vi "Input_Sync_1.vi"(0 "Delay":dbl, 5 "SampClk.Timebase.Rate in":dbl) -> (2 "SampClk.Timebase.Rate 3":dbl, 3 "task out":refnum<k21>, 4 "Refnum out":refnum<k21>, 6 "SampClk.Rate 2":dbl, 8 "error out 2":errorcluster, 10 "FirstSampClkWhen":timestamp, 13 "SampClk.Timebase.Rate out":dbl, 14 "SampClk.Rate":dbl, 15 "error out":errorcluster)   [LabVIEW 2020]
uses:
  <vilib>/DAQmx/create/channels.llb/DAQmx Create Channel (AI-Voltage-Basic).vi
  <vilib>/DAQmx/create/channels.llb/DAQmx Create Channel (TEDS-AI-Voltage-Basic).vi
  <vilib>/DAQmx/configure/timing.llb/DAQmx Timing (Sample Clock).vi
  <vilib>/DAQmx/create/channels.llb/DAQmx Create Channel (AI-Temperature-Thermocouple).vi
  <resource>/objmgr/daqmx.rc
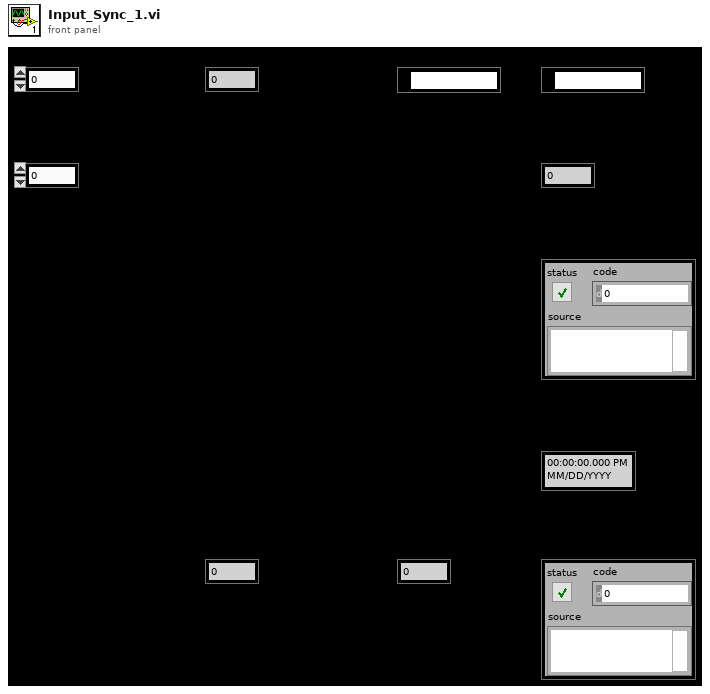
[diagram p1: front panel]
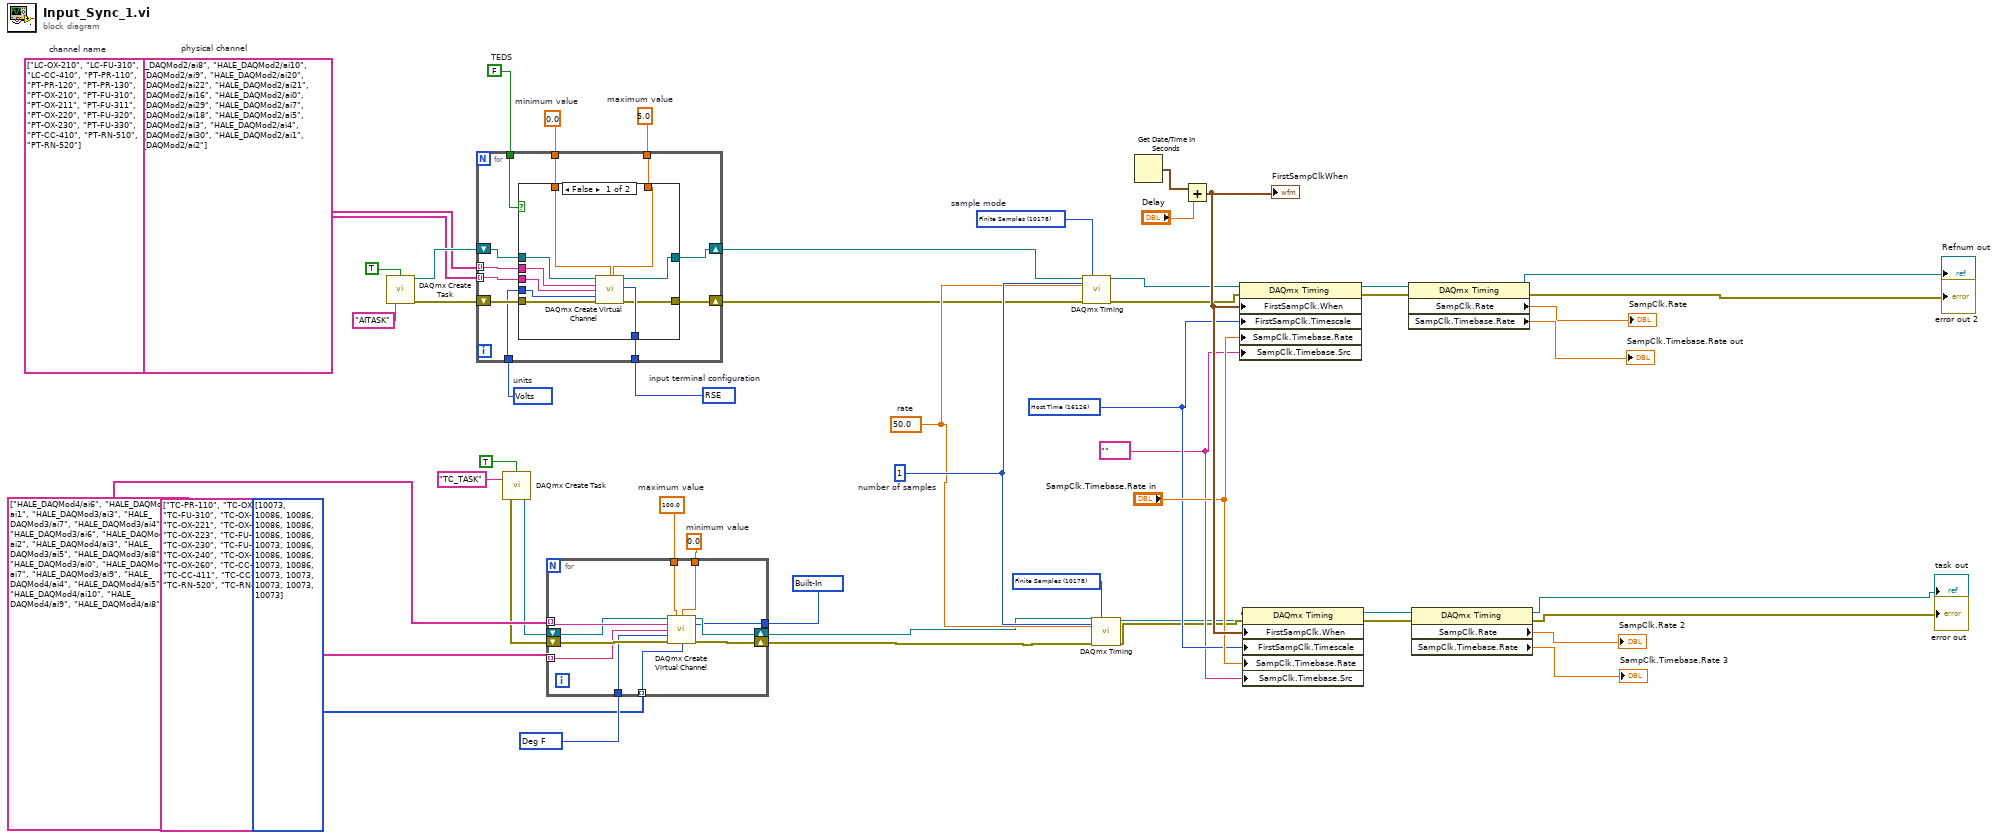
[diagram p0: block diagram]
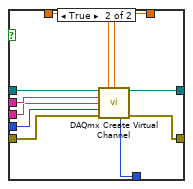
[diagram p2: hidden frame]
diagram:
  w43 = 16126 items=["Host Time"=16126, "I/O Device Time"=16127] ("FirstSampClk.Timescale")
  w39 = tag "" ("SampClk.Timebase.Src")
  w23 = 10200 items=["Built-In"=10200, "Constant Value"=10116, "Channel"=10113] ("cjc source")
  w24 = 0.0  # minimum value
  w25 = 100.0  # maximum value
  w21 = 10144 items=["Deg C"=10143, "Deg F"=10144, "Kelvins"=10325, "Deg R"=10145, "From Custom Scale"=10065] ("units")
  w20 = 10178 items=["Finite Samples"=10178, "Continuous Samples"=10123, "Hardware Timed Single Point"=12522] ("sample mode")
  w15 = i32[] [10073, 10086, 10086, 10086, 10086, 10086, 10086, 10073, 10086, 10086, 10086, 10073, 10086, 10073, 10073, 10073, 10073, 10073] items=["J"=10072, "K"=10073, "N"=10077, "R"=10082, "S"=10085, "T"=10086, "B"=10047, "E"=10055] ("thermocouple type")
  w9 = 5.0  # maximum value
  w10 = 0.0  # minimum value
  w7 = 10178 items=["Finite Samples"=10178, "Continuous Samples"=10123, "Hardware Timed Single Point"=12522]  # sample mode
  w30 = 1  # number of samples
  w29 = 50.0  # rate
  w5 = FALSE  # TEDS
  w3 = 10348 items=["Volts"=10348, "From TEDS"=12516, "From Custom Scale"=10065]  # units
  w8 = string[] ["LC-OX-210", "LC-FU-310", "LC-CC-410", "PT-PR-110", "PT-PR-120", "PT-PR-130", "PT-OX-210", "PT-FU-310", "PT-OX-211", "PT-FU-311", "PT-OX-220", "PT-FU-320", "PT-OX-230", "PT-FU-330", "PT-CC-410", "PT-RN-510", "PT-RN-520"]  # channel name
  w2 = 10083 items=["default"=-1, "RSE"=10083, "NRSE"=10078, "Differential"=10106, "Pseudodifferential"=12529]  # input terminal configuration
  w1 = tag[] ["HALE_DAQMod2/ai8", "HALE_DAQMod2/ai10", "HALE_DAQMod2/ai9", "HALE_DAQMod2/ai20", "HALE_DAQMod2/ai22", "HALE_DAQMod2/ai21", "HALE_DAQMod2/ai16", "HALE_DAQMod2/ai0", "HALE_DAQMod2/ai29", "HALE_DAQMod2/ai7", "HALE_DAQMod2/ai18", "HALE_DAQMod2/ai5", "HALE_DAQMod2/ai3", "HALE_DAQMod2/ai4", "HALE_DAQMod2/ai30", "HALE_DAQMod2/ai1", "HALE_DAQMod2/ai2"]  # physical channel
  n1 = call <vilib>:"DAQmx Create Task.vi"("new task name"="AITASK", "auto cleanup"=TRUE) -> ("task out"=w12:refnum<k21>, "error out"=w14:errorcluster)  [unwired: 12 in]
  n2 = for {
    tunnel: w2 -> [w53]
    tunnel: w10 -> [w62]
    tunnel: w9 -> [w63]
    tunnel: w3 -> [w57]
    tunnel: w8 -> [w59] mode=indexing
    tunnel: w1 -> [w58] mode=indexing
    shift-right: [w60] -> w4
    shift-left: w14 -> [w61]
    tunnel: w5 -> [w56]
    shift-right: [w54] -> w6
    shift-left: w12 -> [w55]
    n3 = case shown="False" w56 {
      tunnel: w63 -> [w73 w79]
      tunnel: w62 -> [w64 w80]
      tunnel: w53 -> [w72 w81]
      tunnel: w61 -> [w71 w83]
      tunnel: [w70 w82] -> w60
      tunnel: w59 -> [w69 w77]
      tunnel: w58 -> [w67 w78]
      tunnel: w57 -> [w68 w76]
      tunnel: w55 -> [w65 w74]
      tunnel: [w66 w75] -> w54
      frame False {
        n4 = call-poly <vilib>:"DAQmx Create Virtual Channel.vi"("task in"=w65, "maximum value"=w73, "minimum value"=w64, "input terminal configuration"=w72, "physical channels"=w67, "name to assign"=w69, "units"=w68, "error in"=w71) -> ("task out"=w66:refnum<k21>, "error out"=w70:errorcluster)  [unwired: 6 in]
      }
      frame True {
        n5 = call-poly <vilib>:"DAQmx Create Virtual Channel.vi"("task in"=w74, "maximum value"=w79, "minimum value"=w80, "input terminal configuration"=w81, "physical channels"=w78, "name to assign"=w77, "units"=w76, "error in"=w83) -> ("task out"=w75:refnum<k21>, "error out"=w82:errorcluster)  [unwired: 6 in]
      }
    }
  }
  n6 = call <vilib>:"DAQmx Create Task.vi"("new task name"="TC_TASK", "auto cleanup"=TRUE) -> ("task out"=w17:refnum<k21>, "error out"=w18:errorcluster)  [unwired: 12 in]
  n7 = for {
    tunnel: tag[] ["HALE_DAQMod4/ai6", "HALE_DAQMod3/ai1", "HALE_DAQMod3/ai3", "HALE_DAQMod3/ai7", "HALE_DAQMod3/ai4", "HALE_DAQMod3/ai6", "HALE_DAQMod3/ai2", "HALE_DAQMod4/ai3", "HALE_DAQMod3/ai5", "HALE_DAQMod3/ai8", "HALE_DAQMod3/ai0", "HALE_DAQMod4/ai7", "HALE_DAQMod3/ai9", "HALE_DAQMod4/ai4", "HALE_DAQMod4/ai5", "HALE_DAQMod4/ai10", "HALE_DAQMod4/ai9", "HALE_DAQMod4/ai8"] ("physical channels") -> [w94] mode=indexing
    tunnel: w15 -> [w93] mode=indexing
    shift-right: [w92] -> w27
    shift-left: w17 -> [w90]
    shift-right: [w91] -> w28
    shift-left: w18 -> [w89]
    tunnel: string[] ["TC-PR-110", "TC-OX-210", "TC-FU-310", "TC-OX-220", "TC-OX-221", "TC-OX-222", "TC-OX-223", "TC-FU-320", "TC-OX-230", "TC-FU-330", "TC-OX-240", "TC-OX-250", "TC-OX-260", "TC-CC-410", "TC-CC-411", "TC-CC-412", "TC-RN-520", "TC-RN-530"] ("name to assign") -> [w88] mode=indexing
    tunnel: w25 -> [w87]
    tunnel: w24 -> [w86]
    tunnel: w23 -> [w85]
    tunnel: w21 -> [w84]
    n8 = call-poly <vilib>:"DAQmx Create Virtual Channel.vi"("task in"=w90, "maximum value"=w87, "minimum value"=w86, "physical channels"=w94, "cjc source"=w85, "name to assign"=w88, "units"=w84, "error in"=w89, "thermocouple type"=w93) -> ("task out"=w92:refnum<k21>, "error out"=w91:errorcluster)  [unwired: 5 in]
  }
  n9 = call-poly <vilib>:"DAQmx Timing.vi"("task/channels in"=w6, "sample mode"=w7, "samples per channel"=w30, "rate"=w29, "error in"=w4) -> ("task out"=w31:refnum<k21>, "error out"=w32:errorcluster)  [unwired: 9 in]
  n10 = call-poly <vilib>:"DAQmx Timing.vi"("task/channels in"=w27, "sample mode"=w20, "samples per channel"=w30, "rate"=w29, "error in"=w28) -> ("task out"=w37:refnum<k21>, "error out"=w38:errorcluster)  [unwired: 9 in]
  n11 = Get Date/Time In Seconds() -> (seconds since 1Jan1904=w46:timestamp)
  n12 = Add(x=w46, y="Delay") -> (x+y=w47:timestamp)
  "FirstSampClkWhen" <- w47
  n13 = property class="DAQmx Timing"(reference=w31, error in=w32, "FirstSampClk.When"=w47, "FirstSampClk.Timescale"=w43, "SampClk.Timebase.Rate"="SampClk.Timebase.Rate in", "SampClk.Timebase.Src"=w39) -> (reference out=w33:refnum<k21>, error out=w34:errorcluster)
  n14 = property class="DAQmx Timing"(reference=w37, error in=w38, "FirstSampClk.When"=w47, "FirstSampClk.Timescale"=w43, "SampClk.Timebase.Rate"="SampClk.Timebase.Rate in", "SampClk.Timebase.Src"=w39) -> (reference out=w35:refnum<k21>, error out=w36:errorcluster)
  n15 = property class="DAQmx Timing"(reference=w33, error in=w34) -> (reference out=→"Refnum out":refnum<k21>, error out=→"error out 2":errorcluster, "SampClk.Rate"=→"SampClk.Rate":dbl, "SampClk.Timebase.Rate"=→"SampClk.Timebase.Rate out":dbl)
  n16 = property class="DAQmx Timing"(reference=w35, error in=w36) -> (reference out=→"task out":refnum<k21>, error out=→"error out":errorcluster, "SampClk.Rate"=→"SampClk.Rate 2":dbl, "SampClk.Timebase.Rate"=→"SampClk.Timebase.Rate 3":dbl)
